vi "UR3_model.vi"() -> ()   [LabVIEW 2024]
panel:
  in  "q":dbl[](array[numeric])
  out "Array":T1(array[cluster])=[{"name"="world", "parent"="", "SE3"="", "qlim"=[], "m"=0.0, "r"=[], "I"=[], "Jm"=0.0, "B"=0.0, "Tc"=[], "G"=0.0}, {"name"="base_link", "parent"="world", "SE3"="()", "qlim"=[], "m"=2.0, "r"=[0.0, 0.0, 0.0], "I"=[0.00305, 0.00305, 0.00562, 0.0, 0.0, 0.0], "Jm"=0.0, "B"=0.0, "Tc"=[0.0, 0.0], "G"=0.0}, {"name"="shoulder_link", "parent"="base_link", "SE3"="(0, 0, 0.1519) ⊕ Rz(q)", "qlim"=[-3.14, 3.14], "m"=0.0, "r"=[0.0, 0.0, 0.0], "I"=[0.00809, 0.00809, 0.00562, 0.0, 0.0, 0.0], "Jm"=0.0, "B"=0.0, "Tc"=[0.0, 0.0], "G"=0.0}, {"name"="upper_arm_link", "parent"="shoulder_link", "SE3"="(0, 0.1198, 0; 0°, 90°, -0°) ⊕ Ry(q)", "qlim"=[-3.14, 3.14], "m"=0.0, "r"=[0.0, 0.0, 0.122], "I"=[0.0217, 0.0217, 0.00962, 0.0, 0.0, 0.0], "Jm"=0.0, "B"=0.0, "Tc"=[0.0, 0.0], "G"=0.0}, {"name"="forearm_link", "parent"="upper_arm_link", "SE3"="(0, -0.0925, 0.2437) ⊕ Ry(q)", "qlim"=[-3.14, 3.14], "m"=0.0, "r"=[0.0, 0.0, 0.107], "I"=[0.00655, 0.00655, 0.00354, 0.0, 0.0, 0.0], "Jm"=0.0, "B"=0.0, "Tc"=[0.0, 0.0], "G"=0.0}, {"name"="wrist_1_link", "parent"="forearm_link", "SE3"="(0, 0, 0.2132; 0°, 90°, -0°) ⊕ Ry(q)", "qlim"=[-3.14, 3.14], "m"=0.0, "r"=[0.0, 0.0851, 0.0], "I"=[0.00208, 0.00208, 0.00225, 0.0, 0.0, 0.0], "Jm"=0.0, "B"=0.0, "Tc"=[0.0, 0.0], "G"=0.0}, {"name"="wrist_2_link", "parent"="wrist_1_link", "SE3"="(0, 0.08505, 0) ⊕ Rz(q)", "qlim"=[-3.14, 3.14], "m"=0.0, "r"=[0.0, 0.0, 0.0853], "I"=[0.00208, 0.00208, 0.00225, 0.0, 0.0, 0.0], "Jm"=0.0, "B"=0.0, "Tc"=[0.0, 0.0], "G"=0.0}, {"name"="wrist_3_link", "parent"="wrist_2_link", "SE3"="(0, 0, 0.08535) ⊕ Ry(q)", "qlim"=[-3.14, 3.14], "m"=0.0, "r"=[0.0, 0.0619, 0.0], "I"=[0.000136, 0.000136, 0.000179, 0.0, 0.0, 0.0], "Jm"=0.0, "B"=0.0, "Tc"=[0.0, 0.0], "G"=0.0}, {"name"="ee_link", "parent"="wrist_3_link", "SE3"="(0, 0.0819, 0; 0°, -0°, 90°)", "qlim"=[], "m"=0.0, "r"=[], "I"=[], "Jm"=0.0, "B"=0.0, "Tc"=[], "G"=0.0}, {"name"="tool0", "parent"="wrist_3_link", "SE3"="(0, 0.0819, 0; -90°, -0°, 0°)", "qlim"=[], "m"=0.0, "r"=[], "I"=[], "Jm"=0.0, "B"=0.0, "Tc"=[], "G"=0.0}, {"name"="base", "parent"="base_link", "SE3"="(0°, -0°, -180°)", "qlim"=[], "m"=0.0, "r"=[], "I"=[], "Jm"=0.0, "B"=0.0, "Tc"=[], "G"=0.0}]
  in  "ur = rtb.models.UR3()":string="Link world: \nLink(\"world\")\nLink base_link: \nLink(\"base_link\", SE3(), parent=\"world\", m=2, r=[0, 0, 0], I=[0.00305, 0.00305, 0.00562, 0, 0, 0], Jm=0, B=0, Tc=[0, 0], G=0)\nLink shoulder_link: \nLink(\"shoulder_link\", SE3(0, 0, 0.1519) ⊕ Rz(q), parent=\"base_link\", qlim=[-3.14, 3.14], m=2, r=[0, 0, 0], I=[0.00809, 0.00809, 0.00562, 0, 0, 0], Jm=0, B=0, Tc=[0, 0], G=0)\nLink upper_arm_link: \nLink(\"upper_arm_link\", SE3(0, 0.1198, 0; 0°, 90°, -0°) ⊕ Ry(q), parent=\"shoulder_link\", qlim=[-3.14, 3.14], m=3.42, r=[0, 0, 0.122], I=[0.0217, 0.0217, 0.00962, 0, 0, 0], Jm=0, B=0, Tc=[0, 0], G=0)\nLink forearm_link: \nLink(\"forearm_link\", SE3(0, -0.0925, 0.2437) ⊕ Ry(q), parent=\"upper_arm_link\", qlim=[-3.14, 3.14], m=1.26, r=[0, 0, 0.107], I=[0.00655, 0.00655, 0.00354, 0, 0, 0], Jm=0, B=0, Tc=[0, 0], G=0)\nLink wrist_1_link: \nLink(\"wrist_1_link\", SE3(0, 0, 0.2132; 0°, 90°, -0°) ⊕ Ry(q), parent=\"forearm_link\", qlim=[-3.14, 3.14], m=0.8, r=[0, 0.0851, 0], I=[0.00208, 0.00208, 0.00225, 0, 0, 0], Jm=0, B=0, Tc=[0, 0], G=0)\nLink wrist_2_link: \nLink(\"wrist_2_link\", SE3(0, 0.08505, 0) ⊕ Rz(q), parent=\"wrist_1_link\", qlim=[-3.14, 3.14], m=0.8, r=[0, 0, 0.0853], I=[0.00208, 0.00208, 0.00225, 0, 0, 0], Jm=0, B=0, Tc=[0, 0], G=0)\nLink wrist_3_link: \nLink(\"wrist_3_link\", SE3(0, 0, 0.08535) ⊕ Ry(q), parent=\"wrist_2_link\", qlim=[-3.14, 3.14], m=0.35, r=[0, 0.0619, 0], I=[0.000136, 0.000136, 0.000179, 0, 0, 0], Jm=0, B=0, Tc=[0, 0], G=0)\nLink ee_link: \nLink(\"ee_link\", SE3(0, 0.0819, 0; 0°, -0°, 90°), parent=\"wrist_3_link\")\nLink tool0: \nLink(\"tool0\", SE3(0, 0.0819, 0; -90°, -0°, 0°), parent=\"wrist_3_link\")\nLink base: \nLink(\"base\", SE3(0°, -0°, -180°), parent=\"base_link\")"
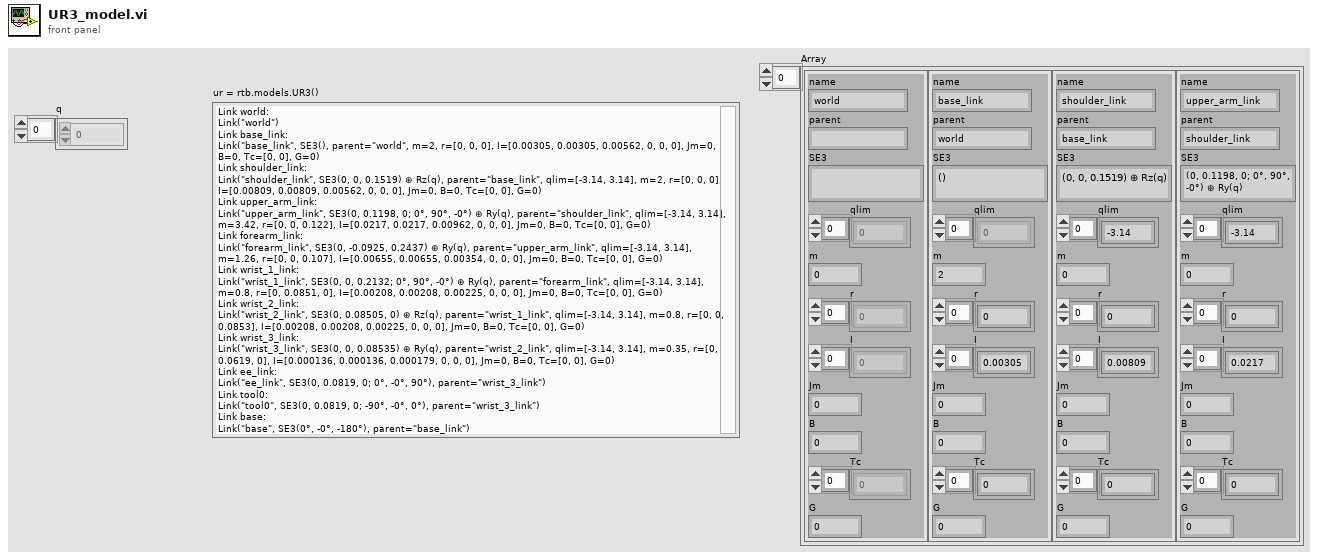
[diagram p1: front panel]
types:
  T1 = cluster{"name":string, "parent":string, "SE3":string, "qlim":dbl[], "m":dbl, "r":dbl[], "I":dbl[], "Jm":dbl, "B":dbl, "Tc":dbl[], "G":dbl}[]
  T2 = cluster{"name":string, "parent":string, "SE3":string, "qlim":dbl[], "m":dbl, "r":dbl[], "I":dbl[], "Jm":dbl, "B":dbl, "Tc":dbl[], "G":dbl}
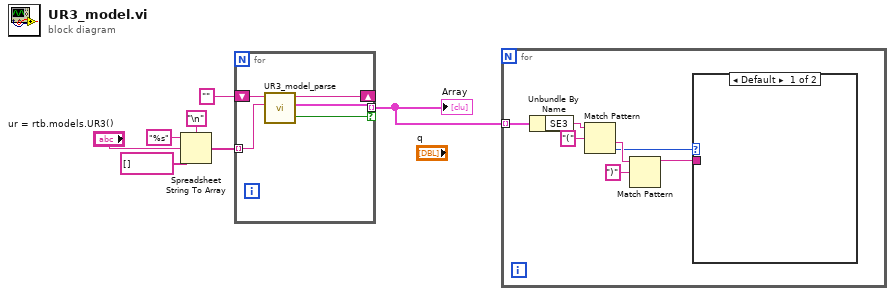
[diagram p0: block diagram]
diagram:
  n1 = Spreadsheet String To Array(delimiter (Tab)="\n", format string="%s", spreadsheet string="ur = rtb.models.UR3()", array type (2D Dbl)=string[] []) -> (array=w3:string[])
  n2 = for {
    tunnel: w3 -> [w12] mode=indexing
    shift-right: [w10] -> _
    shift-left: "" ("trimmed string") -> [w11]
    tunnel: [w9] -> w1 mode=indexing if=w8
    n3 = call "UR3_model_parse.vi"("Link info"=w12, "Name"=w11) -> ("Good point?"=w8:bool, "Info"=w9:T2, "name out"=w10:string)  [unwired: 7 in]
  }
  "Array" <- w1
  n4 = for {
    tunnel: w1 -> [w19] mode=indexing
    n5 = Unbundle By Name(w19) -> ("SE3"=w18:string)
    n6 = Match Pattern(string=w18, regular expression="(") -> (after substring=w15:string, offset past match=w14:i32)  [unwired: 1 in, 2 out]
    n7 = Match Pattern(string=w15, regular expression=")") -> (before substring=w13:string)  [unwired: 1 in, 3 out]
    n8 = case shown="Default" w14 {
      tunnel: w13 -> [_ _]
      frame Default {
      }
      frame -1 {
      }
    }
  }
